vi "Chroma 1905x Series Configure IR Low Limit Query.vi"(7 "Mode":u16(ring) items=["IR"], 8 "error in (no error)":errorcluster, 10 "Step":T1=1 min=1 max=99 step=1, 11 "VISA resource name":refnum<visa-resource-name>) -> (0 "error out":errorcluster, 3 "VISA resource name out":refnum<visa-resource-name>)   [LabVIEW 2025]
uses:
  step--control.ctl
panel:
  out "IR Lo limit value [ohm]":string
  # "IR Low Limit query"
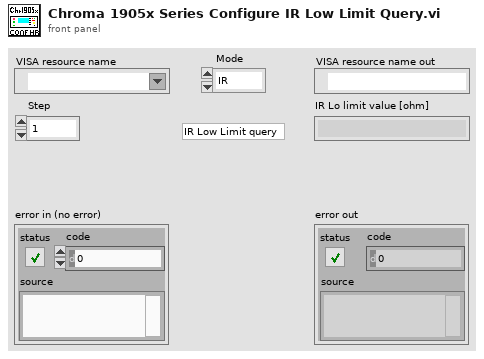
[diagram p1: front panel]
types:
  T1 = typedef "step--control.ctl" = u8
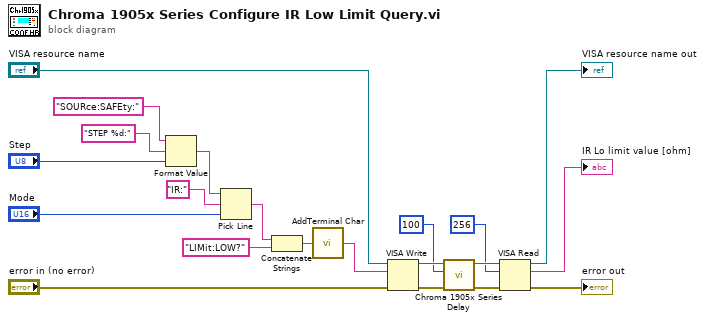
[diagram p0: block diagram]
diagram:
  n1 = Format Value(string ("")="SOURce:SAFEty:", format string="STEP %d:", value (0)="Step") -> (output string=w16:string)
  n2 = Pick Line(string ("")=w16, multi-line string="IR:", line index="Mode") -> (output string=w14:string)
  n3 = Concatenate Strings(w14, "LIMit:LOW?" ("format string")) -> (w13:string)
  n4 = call "AddTerminal Char.vi"("Cmd string"=w13) -> ("Concatenated String"=w3:string)  [unwired: 4 in]
  n5 = VISA Write(VISA resource name="VISA resource name", write buffer=w3, error in (no error)="error in (no error)") -> (VISA resource name out=w10:refnum<visa-resource-name>, error out=w12:errorcluster)  [unwired: 1 out]
  n6 = call "Chroma 1905x Series Delay.vi"("error in (no error)"=w12, "Time Delay [ms]"=u32 100 ("Time Delay ms"), "VISA resource name"=w10) -> ("error out"=w11:errorcluster, "VISA resource name 2"=w9:refnum<visa-resource-name>)  [unwired: 7 in]
  n7 = VISA Read(VISA resource name=w9, byte count=u32 256, error in (no error)=w11) -> (VISA resource name out=→"VISA resource name out":refnum<visa-resource-name>, read buffer=→"IR Lo limit value [ohm]":string, error out=→"error out":errorcluster)  [unwired: 1 out]
